vi "MatrixCalculate.vi"(8 "error in (no error)":errorcluster, 9 "I index":dbl, 10 "xk":dbl[](array[numeric]), 11 "Sync":cdb[](array[numeric])) -> (0 "error out":errorcluster, 3 "output cluster":T1)   [LabVIEW 2014, in "AppPlugins.lvlib" / "ModelValidationPlugin.lvclass"]
uses:
  ModelValidationPlugin.lvclass
  MatrixOutput.ctl
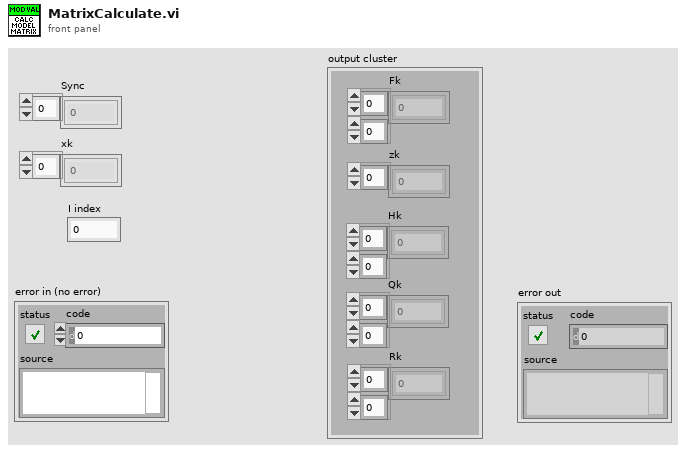
[diagram p1: front panel]
types:
  T1 = typedef "AppPlugins.lvlib/ModelValidationPlugin.lvclass/MatrixOutput.ctl" = cluster{"Fk":dbl[][], "zk":dbl[], "Hk":dbl[][], "Qk":dbl[][], "Rk":dbl[][]}
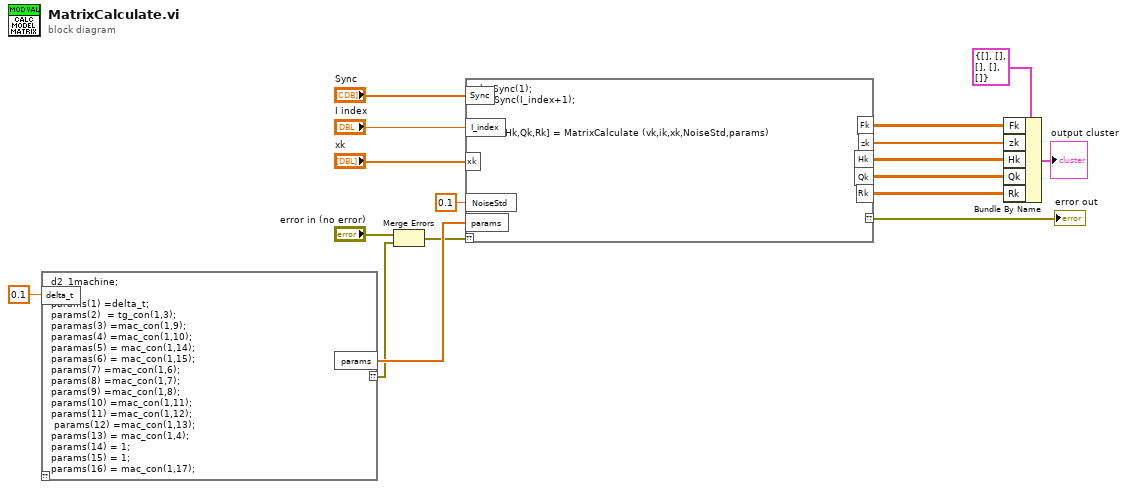
[diagram p0: block diagram]
diagram:
  n1 = script code="d2_1machine;\n\nparams(1) =delta_t;\nparams(2)  = tg_con(1,3);\nparamas(3) =mac_con(1,9);\nparamas(4) =mac_con(1,10);\nparamas(5) = mac_con(1,14);\nparamas(6) = mac_con(1,15);\nparams(7) =mac_con(1,6);\nparams(8) =mac_con(1,7);\nparams(9) =mac_con(1,8);\nparams(10) =mac_con(1,11);\nparams(11) =mac_con(1,12);\n params(12) =mac_con(1,13);\nparams(13) = mac_con(1,4);\nparams(14) = 1;\nparams(15) = 1; \nparams(16) = mac_con(1,17);"("delta_t"=0.1 ("Real")) -> ("??"=w1:errorcluster, "params"=w6:dbl[])  [unwired: 1 in]
  n2 = Merge Errors("error in (no error)", w1) -> (w2:errorcluster)
  n3 = script code="vk=Sync(1);\nik= Sync(I_index+1);\n\n\n[Fk,zk,Hk,Qk,Rk] = MatrixCalculate (vk,ik,xk,NoiseStd,params)"("??"=w2, "Sync"="Sync", "I_index"="I index", "xk"="xk", "NoiseStd"=0.1 ("Real"), "params"=w6) -> ("??"=→"error out":errorcluster, "Fk"=w14:dbl[][], "zk"=w13:dbl[], "Hk"=w12:dbl[][], "Qk"=w11:dbl[][], "Rk"=w10:dbl[][])
  n4 = Bundle By Name(cluster=T1 {"Fk"=[], "zk"=[], "Hk"=[], "Qk"=[], "Rk"=[]} ("MatrixCalculateOutput"), "Fk"=w14, "zk"=w13, "Hk"=w12, "Qk"=w11, "Rk"=w10) -> (→"output cluster":T1)
